vi "process.vi"(8 "error in (no error)":errorcluster, 10 "_data.lvlib:_data.lvclass":refnum<class "_data.lvclass">, 11 "dataTA in":refnum<class "dataTA.lvclass">) -> (0 "error out":errorcluster, 3 "dataTA out":refnum<class "dataTA.lvclass">)   [LabVIEW 2019, in "dataTA.lvlib" / "dataTA.lvclass"]
uses:
  dataTA.lvclass
  _data/_data.lvlibp/_dataClass/_data.lvclass
  dataTA.lvclass/dataTA.ctl
  <vilib>/Analysis/NI_AALBase.lvlib
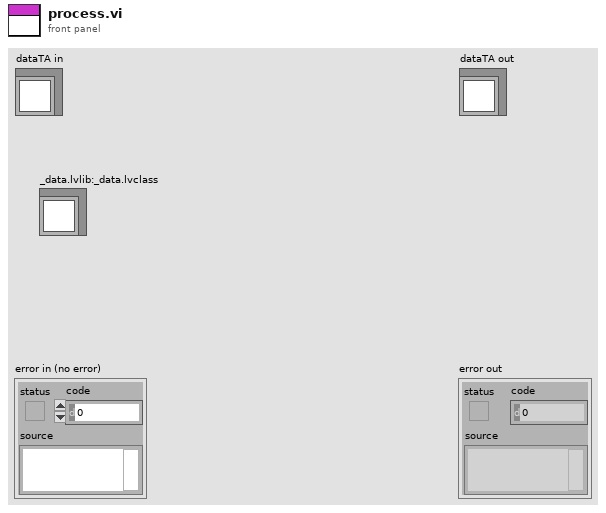
[diagram p1: front panel]
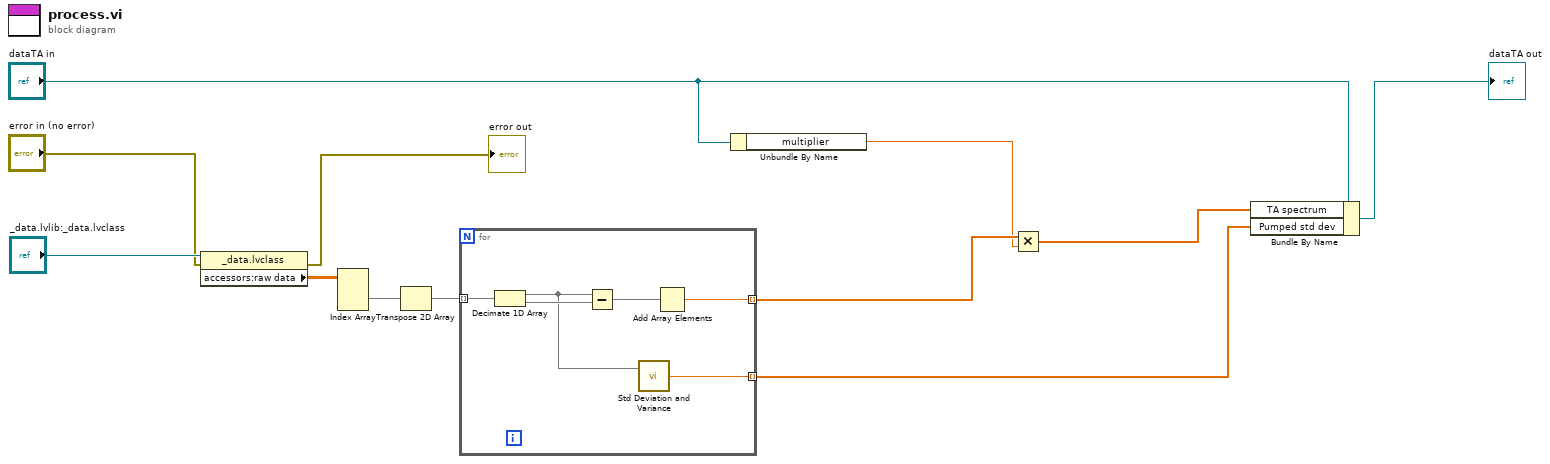
[diagram p0: block diagram]
diagram:
  n1 = property class="_data.lvclass"(reference="_data.lvlib:_data.lvclass", error in="error in (no error)") -> (error out=→"error out":errorcluster, "accessors:raw data"=w10:dbl[][][])  [unwired: 1 out]
  n2 = Index Array(array=w10) -> (element=w9:dbl[][])  [unwired: 3 in]
  n3 = Transpose 2D Array(2D array=w9) -> (transposed array=w6:dbl[][])
  n4 = for {
    tunnel: w6 -> [w18] mode=indexing
    tunnel: [w15] -> w3 mode=indexing
    tunnel: [w13] -> w5 mode=indexing
    n5 = Decimate 1D Array(w18) -> (w14:dbl[], w17:dbl[])
    n6 = Subtract(x=w14, y=w17) -> (x-y=w16:dbl[])
    n7 = call <vilib>:"Std Deviation and Variance.vi"("X"=w14) -> ("standard deviation"=w13:dbl)  [unwired: 1 in, 2 out]
    n8 = Add Array Elements(numeric array=w16) -> (sum=w15:dbl)
  }
  n9 = Unbundle By Name("dataTA in") -> ("multiplier"=w2:dbl)
  n10 = Multiply(x=w3, y=w2) -> (x*y=w1:dbl[])
  n11 = Bundle By Name(cluster="dataTA in", "TA spectrum"=w1, "Pumped std dev"=w5) -> (→"dataTA out":refnum<class "dataTA.lvclass">)
